vi "my UDP Receiver.vi"() -> ()   [LabVIEW 2014]
panel:
  out "数组":dbl[][](array[numeric])
  in  "停止":bool
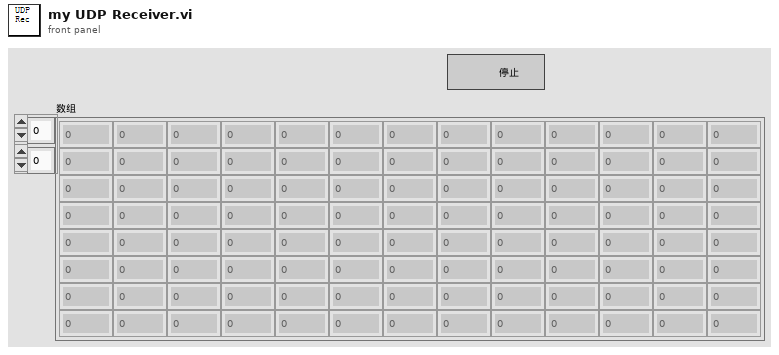
[diagram p1: front panel]
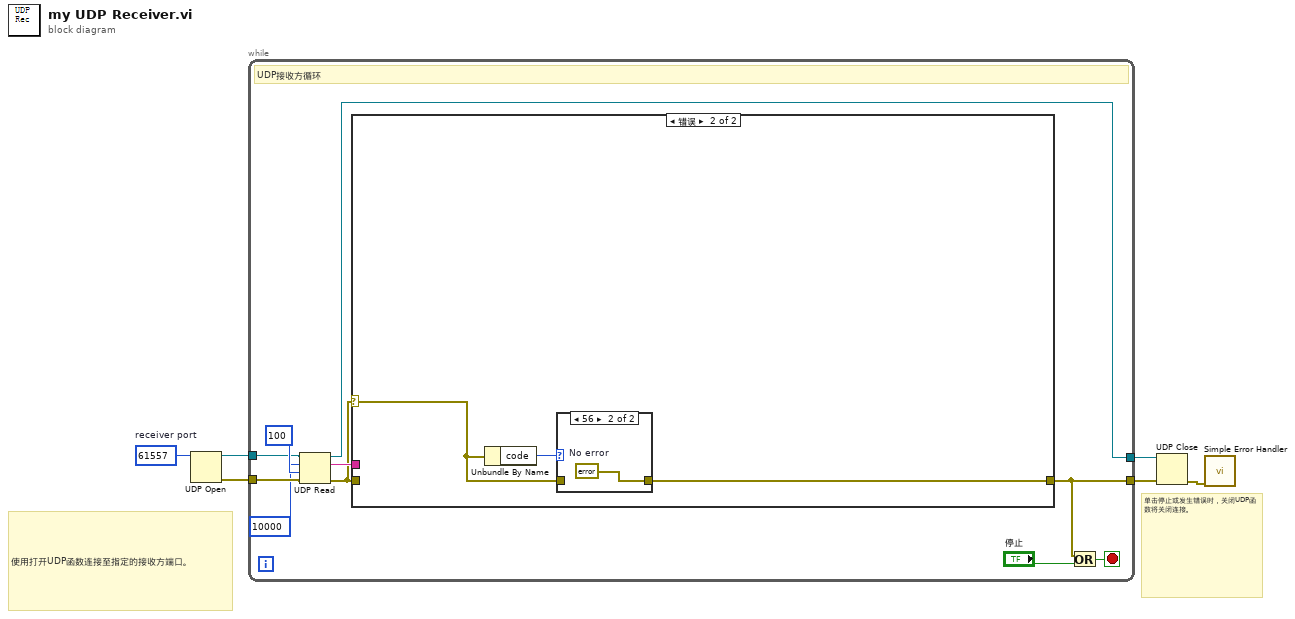
[diagram p0: block diagram]
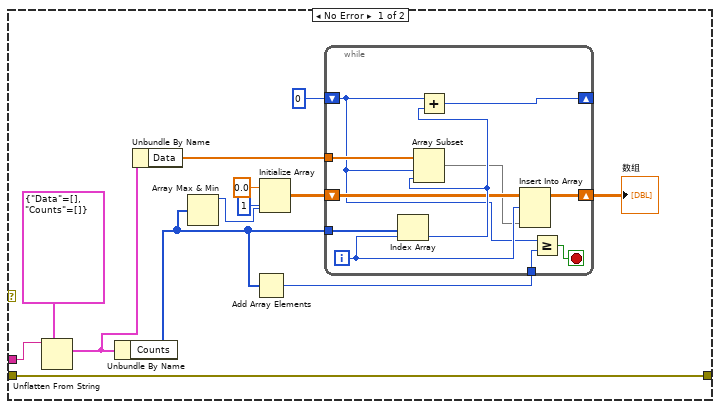
[diagram p2: hidden frame]
diagram:
  w4 = u16 61557  # receiver port
  # "单击停止或发生错误时，关闭UDP函数将关闭连接。"
  # "使用打开UDP函数连接至指定的接收方端口。"
  n1 = UDP Open(11:w4) -> (port=w2:refnum<k16>, 0:w1:errorcluster)  [unwired: 4 in, 1 out]
  n2 = while {
    tunnel: [w12] -> w6
    tunnel: [w9] -> w3
    tunnel: w1 -> [w11]
    tunnel: w2 -> [w10]
    stop <- w15 stop-if-true
    # "UDP接收方循环"
    n3 = UDP Read(connection ID=w10, max size (548)=10000 ("最大值(548)"), timeout ms (25000)=100, 8:w11) -> (data out=w13:string, error out=w8:errorcluster, 3:w12:refnum<k16>)  [unwired: 2 out]
    n4 = case shown="错误" w8 {
      selector: w8 -> [_ w42]
      tunnel: w13 -> [w27 _]
      tunnel: [w28 w41] -> w9
      tunnel: w8 -> [w28 _]
      frame No Error {
        # "发送方发送了数据。更新图表值。"
        n5 = Unflatten From String(type=cluster{"Data":dbl[], "Counts":i32[]} {"Data"=[], "Counts"=[]}, binary string=w27) -> (value=w19:cluster{"Data":dbl[], "Counts":i32[]})  [unwired: 3 in, 2 out]
        n6 = Unbundle By Name(w19) -> ("Counts"=w20:i32[])
        n7 = Unbundle By Name(w19) -> ("Data"=w18:dbl[])
        n8 = Array Max & Min(array=w20) -> (max value=w21:i32)  [unwired: 3 out]
        n9 = Add Array Elements(numeric array=w20) -> (sum=w23:i32)
        n10 = Initialize Array(0.0 ("元素"), 1 ("维数大小"), w21) -> (w24:dbl[][])
        n11 = while {
          shift-right: [w39] -> _
          shift-left: 0 -> [w30]
          tunnel: w18 -> [w40]
          shift-right: [w37] -> w17
          shift-left: w24 -> [w36]
          tunnel: w20 -> [w33]
          tunnel: w23 -> [w31]
          i -> [w35]
          stop <- w32 stop-if-true
          n12 = Index Array(array=w33, index=w35) -> (element=w38:i32)
          n13 = Array Subset(array=w40, index=w30, length=w38) -> (w34:dbl[])
          n14 = Add(x=w30, y=w38) -> (x+y=w39:i32)
          n15 = Insert Into Array(array=w36, index (row)=w35, new element=w34) -> (w37:dbl[][])  [unwired: 1 in]
          n16 = Greater Or Equal?(x=w30, y=w31) -> (x >= y?=w32:bool)
        }
        "数组" <- w17
      }
      frame Error {
        # "发送方未发送数据。忽略超时错误并继续等待。"
        n17 = Unbundle By Name(w42) -> ("code"=w43:i32)
        n18 = case shown="56" w43 {
          tunnel: w42 -> [w44 _]
          tunnel: [w44 w45] -> w41
          frame Default {
          }
          frame 56 {
            w45 = errorcluster {"status"=FALSE, "code"=0, "source"=""}  # No error
          }
        }
      }
    }
    n19 = Or(x=w9, y="停止") -> (x .or. y?=w15:bool)
  }
  n20 = UDP Close(connection ID=w6, 8:w3) -> (error out=w5:errorcluster)  [unwired: 1 out]
  n21 = call <vilib>:"Simple Error Handler.vi"("error in (no error)"=w5) -> ()  [unwired: 1 in, 8 out]
